vi "OpeningScreen.vi"() -> ()   [LabVIEW 2017]
doc: "Vi criada para mostrar uma tela inicial para o usuário antes da partida - menu de jogo"
panel:
  in  "Sair do Jogo":bool
  in  "Melhores Pontuações":bool
  in  "Histórico de Partidas":bool
  in  "Informações do App":bool
  in  "Instruções":bool
  in  "Novo Jogo":bool
  # "Bem Vindo!!"
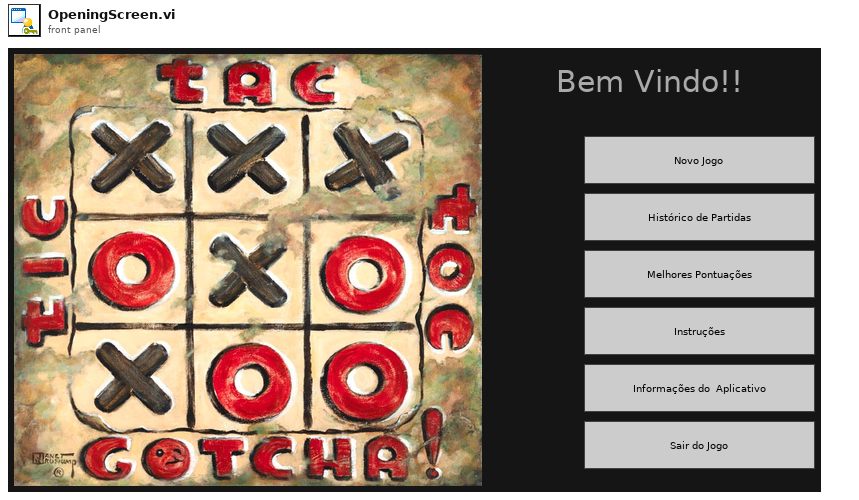
[diagram p1: front panel]
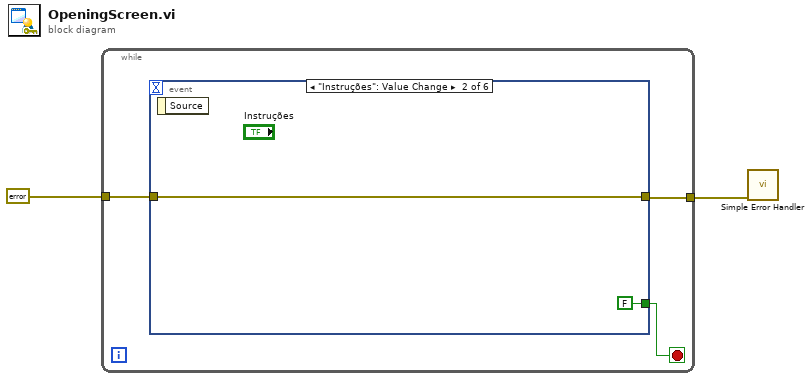
[diagram p0: block diagram]
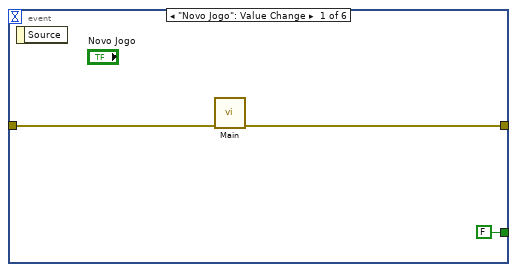
[diagram p2: hidden frame]
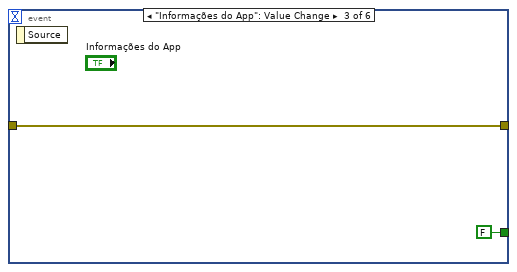
[diagram p3: hidden frame]
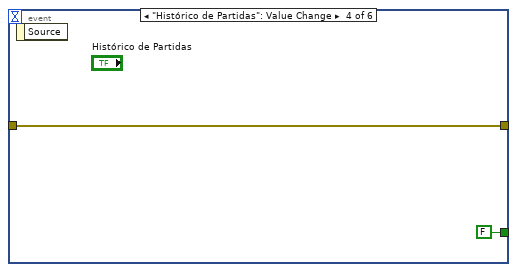
[diagram p4: hidden frame]
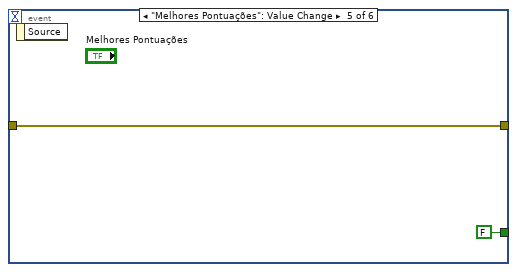
[diagram p5: hidden frame]
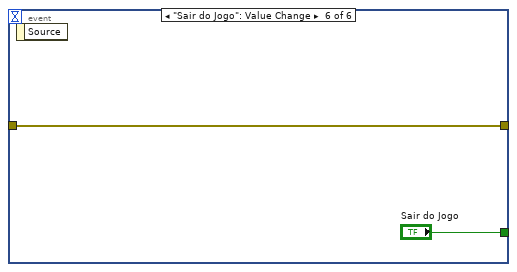
[diagram p6: hidden frame]
diagram:
  n1 = while {
    tunnel: errorcluster {"status"=FALSE, "code"=0, "source"=""} ("error constant") -> [w4]
    tunnel: [w3] -> w1
    stop <- w5 stop-if-true
    n2 = event shown="[1] \"Instruções\": Value Change" {
      selector: _ -> [_ _ _ _ _ _]
      dyn-events: _ -> [_ _ _ _ _ _]
      timeout: _ -> [_ _ _ _ _ _]
      tunnel: [FALSE ("Sair do Jogo") FALSE ("Sair do Jogo") FALSE ("Sair do Jogo") FALSE ("Sair do Jogo") FALSE ("Sair do Jogo") "Sair do Jogo"] -> w5
      tunnel: w4 -> [w7 w9 w11 w13 w15 w17]
      tunnel: [w6 w9 w11 w13 w15 w17] -> w3
      event "Novo Jogo": Value Change {
        n3 = event-data() -> ()  [unwired: 1 in, 1 out]
        n4 = call "Main.vi"("Error In"=w7) -> ("Error Out"=w6:errorcluster)  [unwired: 10 in]
      }
      event "Instruções": Value Change {
        n5 = event-data() -> ()  [unwired: 1 in, 1 out]
      }
      event "Informações do App": Value Change {
        n6 = event-data() -> ()  [unwired: 1 in, 1 out]
      }
      event "Histórico de Partidas": Value Change {
        n7 = event-data() -> ()  [unwired: 1 in, 1 out]
      }
      event "Melhores Pontuações": Value Change {
        n8 = event-data() -> ()  [unwired: 1 in, 1 out]
      }
      event "Sair do Jogo": Value Change {
        n9 = event-data() -> ()  [unwired: 1 in, 1 out]
      }
    }
  }
  n10 = call <vilib>:"Simple Error Handler.vi"("error in (no error)"=w1) -> ()  [unwired: 4 in, 5 out]
